vi "Delay Groupdata inquiry.vi"(8 "error in (no error)":errorcluster, 11 "VISA resource name":refnum<visa-resource-name>) -> (0 "error out":errorcluster, 1 "Time Set":string, 2 "Pattern":string, 3 "VISA resource name out":refnum<visa-resource-name>)   [LabVIEW 2020, in "GPP.lvlib"]
uses:
  GPP.lvlib
  Function/VISA_COMMON.ctl
panel:
  in  "Channel  (1: CH1)":u16(ring)=1 items=["CH1"=1, "CH2"=2, "CH3"=3, "CH4"=4]
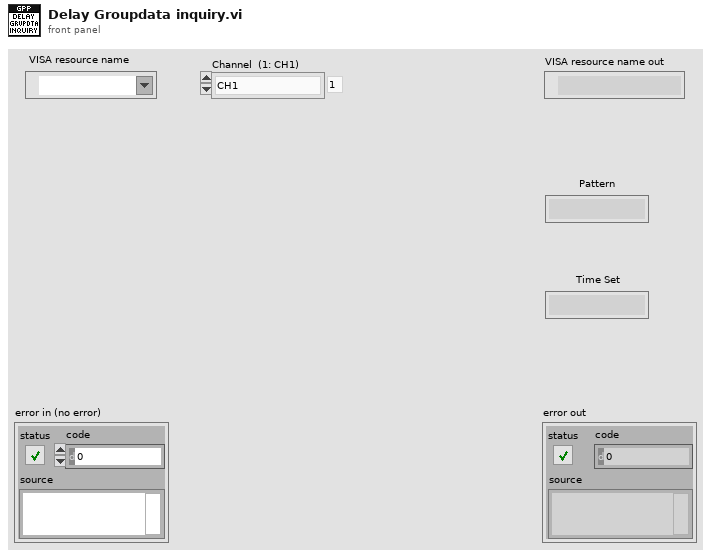
[diagram p1: front panel]
types:
  T1 = typedef "GPP.lvlib/VISA_COMMON.ctl" = enum16{"Initial", "Write CMD", "Read Result", "Read History", "Close"}
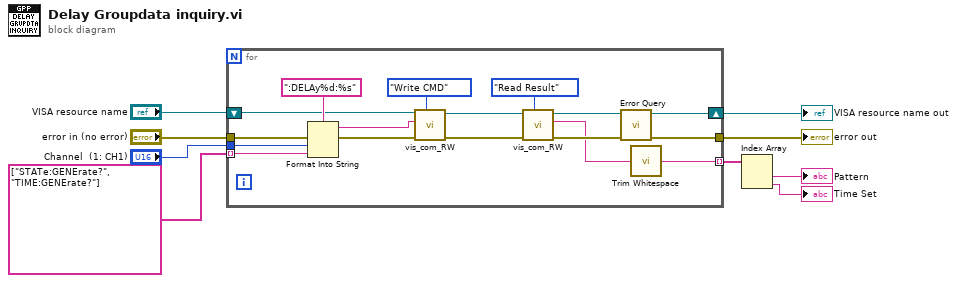
[diagram p0: block diagram]
diagram:
  n1 = for {
    tunnel: "error in (no error)" -> [w20]
    tunnel: "Channel  (1: CH1)" -> [w18]
    tunnel: string[] ["STATe:GENErate?", "TIME:GENErate?"] -> [w15] mode=indexing
    tunnel: [w16] -> w4
    tunnel: [w12] -> w6 mode=indexing
    shift-right: [w10] -> w3
    shift-left: "VISA resource name" -> [w14]
    n2 = Format Into String(format string=":DELAy%d:%s", error in=w20, w18, w15) -> (resulting string=w13:string, error out=w19:errorcluster)  [unwired: 1 in]
    n3 = call "vis_com_RW.vi"("Funciton"=VISA_COMMON."Write CMD", "error in (no error)"=w19, "CMD String"=w13, "VISA resource in"=w14) -> ("error out"=w24:errorcluster, "VISA resource out"=w23:refnum<visa-resource-name>)  [unwired: 5 in, 1 out]
    n4 = call "vis_com_RW.vi"("Funciton"=VISA_COMMON."Read Result", "error in (no error)"=w24, "VISA resource in"=w23) -> ("error out"=w21:errorcluster, "Result"=w11:string, "VISA resource out"=w22:refnum<visa-resource-name>)  [unwired: 6 in]
    n5 = call "Error Query.vi"("error in (no error)"=w21, "VISA resource name"=w22) -> ("error out"=w16:errorcluster, "VISA resource name out"=w10:refnum<visa-resource-name>)  [unwired: 6 in, 2 out]
    n6 = call <vilib>:"Trim Whitespace.vi"("string"=w11) -> ("trimmed string"=w12:string)  [unwired: 1 in]
  }
  "error out" <- w4
  "VISA resource name out" <- w3
  n7 = Index Array(array=w6) -> (element #1=→"Pattern":string, element #2=→"Time Set":string)  [unwired: 2 in]
